vi "SecurityAcess SendKey.vi"(5 "LogSuspend":bool, 8 "error in":errorcluster, 10 "Key":string, 11 "UdsHandleIn":T1={"LogPath"=path "", "LogEnabled"=FALSE, "isOpen"=FALSE, "LogContent"="", "Adapter"="CAN0", "MCanHandle"={"MCanAdapter"=refnum}, "TransmittId"=0, "ReceiveId"=0}) -> (0 "error out":errorcluster, 3 "UdsHandleOut":T1={"LogPath"=path "", "LogEnabled"=FALSE, "isOpen"=FALSE, "LogContent"="", "Adapter"="CAN0", "MCanHandle"={"MCanAdapter"=refnum}, "TransmittId"=0, "ReceiveId"=0})   [LabVIEW 2011, in "Konvolucio MUDS150628.lvlib"]
uses:
  <instrlib>/Konvolucio MUDS150628/Konvolucio MUDS150628.lvlib
  <instrlib>/Konvolucio MUDS150628/Types/UdsHandleType.ctl
  <instrlib>/Konvolucio MCAN120803/Types/MCanHandleType.ctl
  C:/Program Files/National Instruments/LabVIEW 2011/instr.lib/Konvolucio MCAN120803/Private/Konvolucio.MCAN120803.dll
  Konvolucio MCAN120803/Private/Konvolucio.MCAN120803.dll
  <instrlib>/Konvolucio MCAN120803/Konvolucio MCAN120803.lvlib
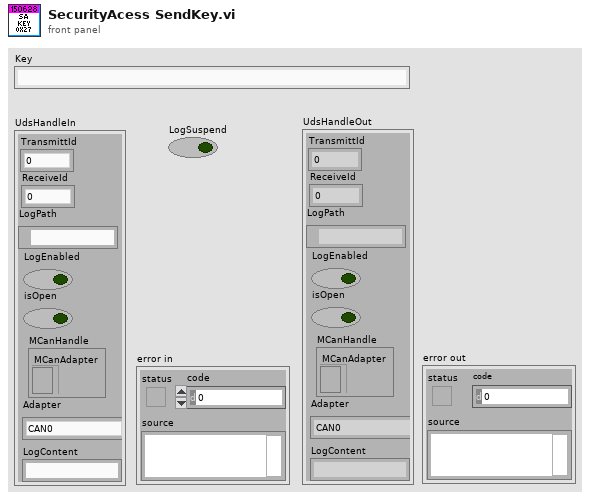
[diagram p1: front panel]
types:
  T1 = typedef "Konvolucio MUDS150628.lvlib/UdsHandleType.ctl" = cluster{"LogPath":path, "LogEnabled":bool, "isOpen":bool, "LogContent":string, "Adapter":string, "MCanHandle":T2, "TransmittId":u32, "ReceiveId":u32}
  T2 = typedef "Konvolucio MCAN120803.lvlib/MCanHandleType.ctl" = cluster{"MCanAdapter":refnum<k24>}
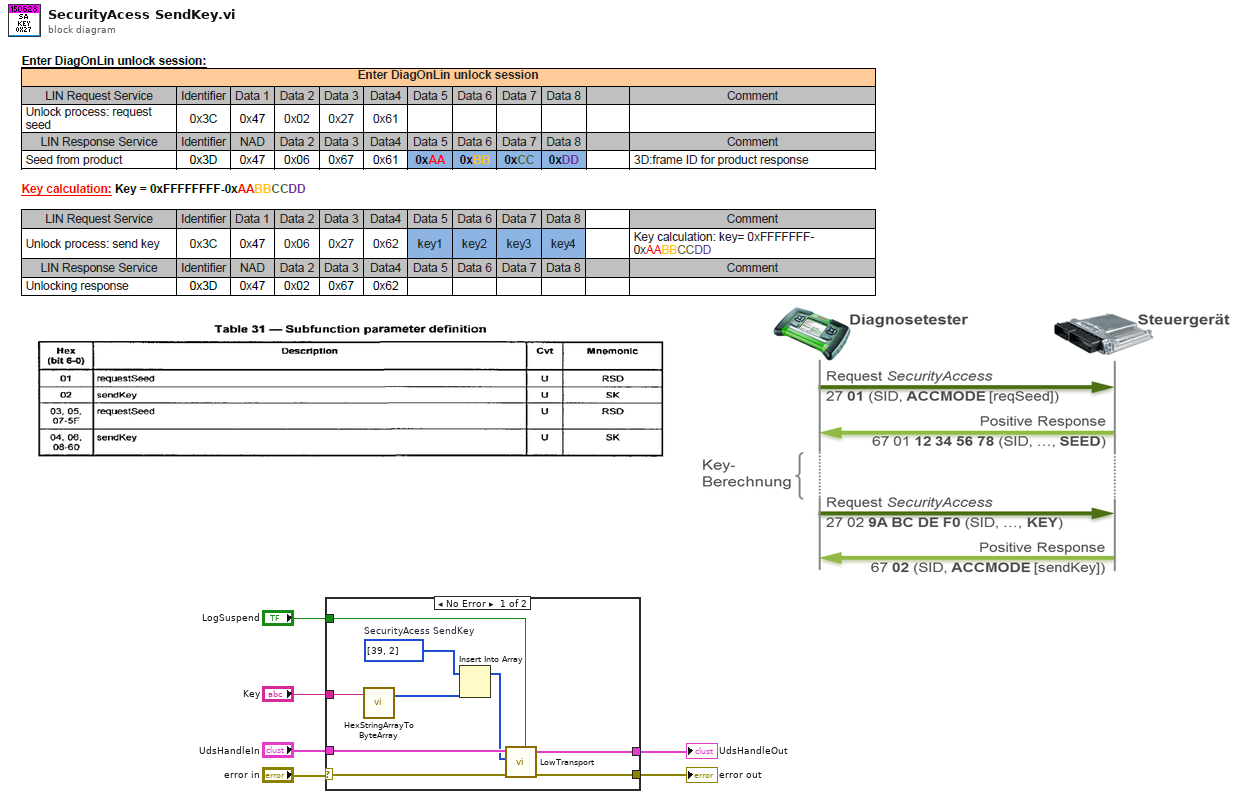
[diagram p0: block diagram]
diagram:
  n1 = case shown="No Error" "error in" {
    selector: "error in" -> [w14 w17]
    tunnel: "UdsHandleIn" -> [w15 w16]
    tunnel: [w13 w17] -> w4
    tunnel: [w12 w16] -> w3
    tunnel: "LogSuspend" -> [w11 _]
    tunnel: "Key" -> [w8 _]
    frame No Error {
      w10 = u8[] [39, 2]  # SecurityAcess SendKey
      n2 = call <instrlib>:"HexStringArrayToByteArray.vi"("HexStirngArray"=w8) -> ("ByteArrayOut"=w7:u8[])  [unwired: 2 in]
      n3 = Insert Into Array(array=w10, new element=w7) -> (w9:u8[])  [unwired: 1 in]
      n4 = call <instrlib>:"LowTransport.vi"("LogSuspend"=w11, "error in"=w14, "Request"=w9, "HandleIn"=w15) -> ("error out"=w13:errorcluster, "HandleOut"=w12:T1)  [unwired: 5 in, 1 out]
    }
    frame Error {
    }
  }
  "error out" <- w4
  "UdsHandleOut" <- w3
